vi "VARIABLE_GLOBAL1.vi"() -> ()   [LabVIEW 2017]
panel:
  out "Numeric 2":dbl
  in  "Numeric":dbl
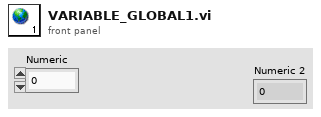
[diagram p1: front panel]
diagram:
